vi "Bind Controls to SmartDashboard.vi"(4 "RPC ref":refnum<user-event>, 6 "Update Time (ms)":i32=100, 8 "Client Name":string="Dashboard", 9 "Path Prefix":string="SmartDashboard", 10 "Bound Control Refs":refnum<vi>[](array[refnum]), 11 "Server IP Address":string="localhost") -> ()   [LabVIEW 2017]
doc: "Place this VI in the Dashboard or other client applications so that it can run in parallel with the other tasks. Provide the robot IP address so that it can know where to find the server. This starts the NT Client automatically.\n\nCombine the path prefix and control name to construct entry names. Bind controls and indicators to a SmartDashboard or Network Table entry with the matching name. Controls and Indicators will be updated each time the table entriy of the same name changes. Table entries will be updated each time the control changes value."
uses:
  <vilib>/Rock Robotics/Network Tables/NT Event Type.ctl
  <vilib>/Rock Robotics/Network Tables/Protocol Operations.ctl
  <vilib>/Rock Robotics/Network Tables/Field Data.ctl
  <vilib>/Rock Robotics/Network Tables/Field Type.ctl
  <vilib>/Rock Robotics/Network Tables/Sequence.ctl
  <vilib>/Rock Robotics/Network Tables/NT Globals.vi
  <vilib>/Rock Robotics/WPI/Dashboard/WPI_DashboardLogging Global.vi
panel:
  in  "Finish":bool
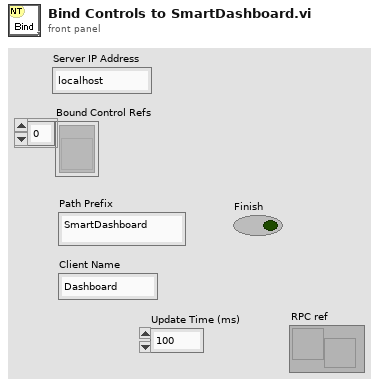
[diagram p1: front panel]
types:
  T1 = typedef "NT Event Type.ctl" = cluster{"Operation":T2, "Name":string, "Field Value":T3}
  T2 = typedef "Protocol Operations.ctl" = enum16{"Unknown", "Keep Alive", "Client Hello", "Version not supported", "Server Hello Complete", "Assign", "Update", "No Op", "Server Hello", "Client Hello Complete", "Update Flags", "Delete Entry", "Delete All", "RPC Exec", "RPC Response"}
  T3 = typedef "Field Data.ctl" = cluster{"Dbl":dbl, "String":string, "Type":T4, "Boolean":bool, "Sequence #":T5, "Flags":u8}
  T4 = typedef "Field Type.ctl" = enum8{"Invalid", "Bool", "Numeric", "String", "Raw", "Boolean Array", "Numeric Array", "String Array", "RPC"}
  T5 = typedef "Sequence.ctl" = u16
  T6 = cluster{"Operation":T2, "Name":string, "Field Value":T3}
  T7 = cluster{cluster{"RPC field ID":u16, "Unique ID":u16}, "String":string}
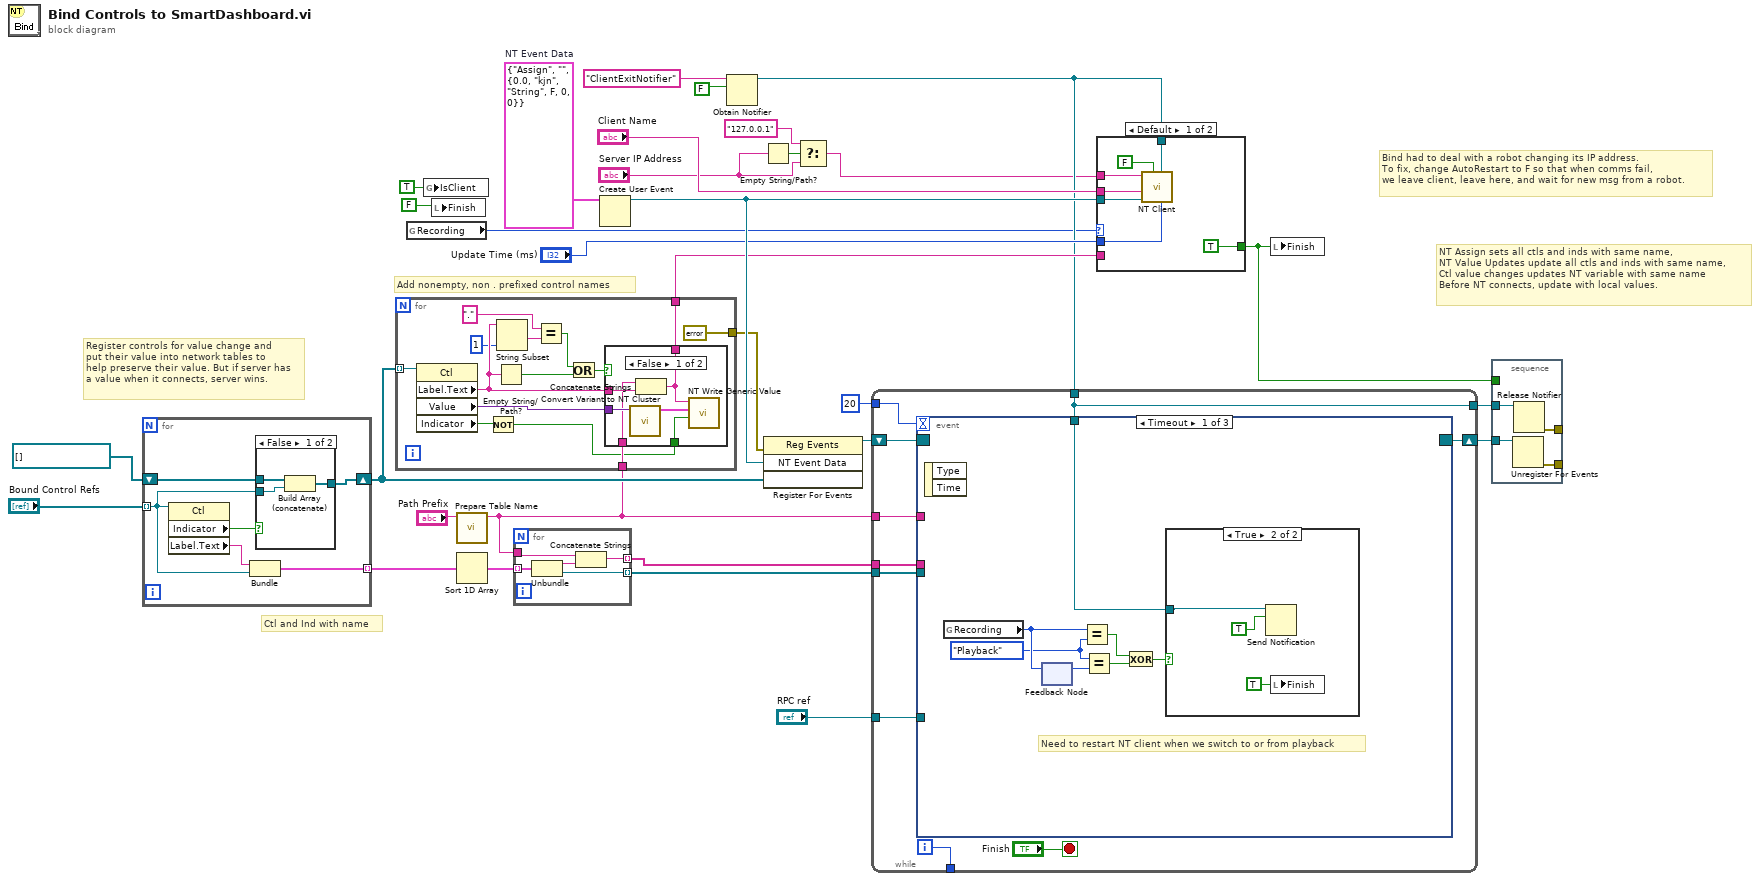
[diagram p0: block diagram]
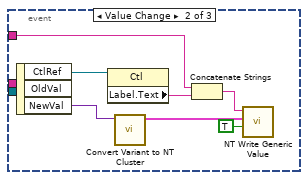
[diagram p3: hidden frame]
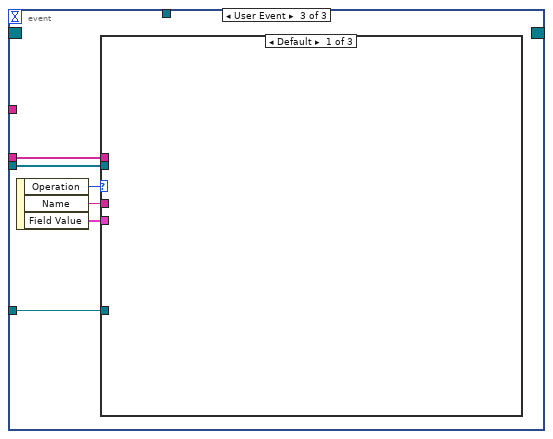
[diagram p4: hidden frame]
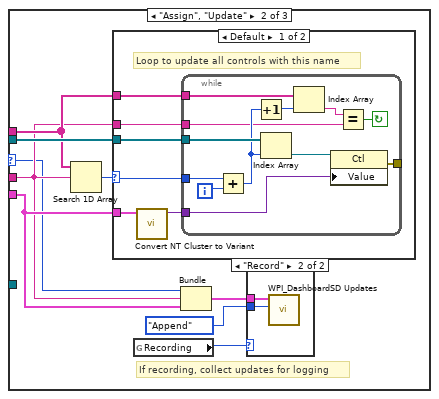
[diagram p5: hidden frame]
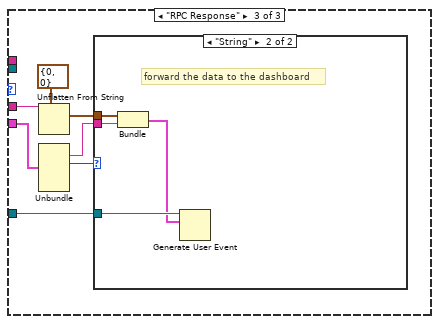
[diagram p8: hidden frame]
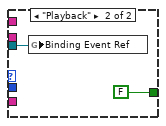
[diagram p10: hidden frame]
diagram:
  w14 = T1 {"Operation"=enum."Assign", "Name"="", "Field Value"={"Dbl"=0.0, "String"="kjn", "Type"=enum."String", "Boolean"=FALSE, "Sequence #"=0, "Flags"=0}}  # NT Event Data
  # "Add nonempty, non . prefixed control names"
  # "Bind had to deal with a robot changing its IP address.\nTo fix, change AutoRestart to F so that when comms fail,\nwe leave client, leave here, and wait for new msg from a robot."
  # "Register controls for value change and\nput their value into network tables to\nhelp preserve their value. But if server has\na value when it connects, server wins."
  # "Ctl and Ind with name"
  # "NT Assign sets all ctls and inds with same name,\nNT Value Updates update all ctls and inds with same name,\nCtl value changes updates NT variable with same name\nBefore NT connects, update with local values."
  n1 = for {
    tunnel: "Bound Control Refs" -> [w34] mode=indexing
    shift-right: [w35] -> w23
    shift-left: refnum<vi>[] [] -> [w36]
    tunnel: [w32] -> w29 mode=indexing
    n2 = property class="Ctl"(reference=w34) -> ("Indicator"=w37:bool, "Label.Text"=w33:string)  [unwired: 1 in, 2 out]
    n3 = Bundle("Label.Text"=w33, w34) -> (w32:cluster{"Label.Text":string, refnum<vi>})  [unwired: 1 in]
    n4 = case shown="False" w37 {
      tunnel: w34 -> [w40 _]
      tunnel: w36 -> [w39 w41]
      tunnel: [w38 w41] -> w35
      frame False {
        n5 = Build Array (concatenate)(w39, w40) -> (w38:refnum<vi>[])
      }
      frame True {
      }
    }
  }
  n6 = global read "WPI_DashboardLogging Global.vi" "Recording"() -> (w3:enum32{"Stop", "Record", "Playback"})
  n7 = global write "NT Globals.vi" "IsClient"(TRUE ("IsClient")) -> ()
  n8 = local write "Finish"(FALSE ("Automatic restart")) -> ()
  n9 = call <vilib>:"Prepare Table Name.vi"("Table Prefix"="Path Prefix") -> ("Prefixed Name"=w21:string)  [unwired: 10 in]
  n10 = for {
    tunnel: w23 -> [w55] mode=indexing
    tunnel: [w53] -> w24
    tunnel: w21 -> [w52]
    tunnel: [errorcluster {"status"=FALSE, "code"=0, "source"=""} ("error out")] -> w1
    n11 = property class="Ctl"(reference=w55) -> ("Label.Text"=w50:string, "Value"=w54:variant, "Indicator"=w43:bool)  [unwired: 1 in, 2 out]
    n12 = Not(x=w43) -> (.not. x?=w42:bool)
    n13 = Empty String/Path?(string/path=w50) -> (empty?=w51:bool)
    n14 = String Subset(string=w50, length (rest)=1) -> (substring=w48:string)  [unwired: 1 in]
    n15 = Equal?(x=".", y=w48) -> (x = y?=w46:bool)
    n16 = Or(x=w46, y=w51) -> (x .or. y?=w45:bool)
    n17 = case shown="False" w45 {
      tunnel: w54 -> [w60 _]
      tunnel: w50 -> [w59 _]
      tunnel: [w58 _] -> w53
      tunnel: w52 -> [w57 _]
      tunnel: w42 -> [w56 _]
      frame False {
        n18 = call <vilib>:"Convert Variant to NT Cluster.vi"("NewVal"=w60) -> ("Field Value"=w61:T3)  [unwired: 10 in]
        n19 = Concatenate Strings(w57, w59) -> (w58:string)
        n20 = call <vilib>:"NT Write Generic Value.vi"("Owning Write"=w56, "Field Value"=w61, "Name"=w58) -> ()  [unwired: 8 in, 1 out]
      }
      frame True {
      }
    }
  }
  n21 = Sort 1D Array(array=w29) -> (sorted array=w28:cluster{"Label.Text":string, refnum<vi>}[])
  n22 = for {
    tunnel: w28 -> [w66] mode=indexing
    tunnel: [w63] -> w27 mode=indexing
    tunnel: [w65] -> w26 mode=indexing
    tunnel: w21 -> [w62]
    n23 = Unbundle(w66) -> ("Label.Text"=w64:string, w65:refnum<vi>)
    n24 = Concatenate Strings(w62, w64) -> (w63:string)
  }
  n25 = Create User Event(user event datatype=w14) -> (user event=w30:refnum<user-event>)  [unwired: 1 in, 1 out]
  n26 = Obtain Notifier(name (unnamed)="ClientExitNotifier", notification data type=FALSE ("Automatic restart")) -> (notifier out=w10:refnum<notifier>)  [unwired: 2 in, 2 out]
  n27 = Empty String/Path?(string/path="Server IP Address") -> (empty?=w8:bool)
  n28 = register-events(error in=w1, w30, w23) -> (reference out=w19:refnum<event-registration>)  [unwired: 1 in, 1 out]
  n29 = Select(t="127.0.0.1" ("name (unnamed)"), s=w8, f="Server IP Address") -> (s? t:f=w7:string)
  n30 = while {
    tunnel: w27 -> [w75]
    tunnel: w26 -> [w74]
    tunnel: w21 -> [w73]
    tunnel: [w72] -> _
    shift-right: [w70] -> w17
    shift-left: w19 -> [w71]
    tunnel: w10 -> [w69]
    tunnel: [w69] -> w11
    tunnel: 20 -> [w68]
    tunnel: "RPC ref" -> [w67]
    i -> [w72]
    stop <- "Finish" stop-if-true
    n31 = event shown="[0] Timeout" {
      selector: w71 -> [_ _ _]
      dyn-events: [_ _ _] -> w70
      timeout: w68 -> [_ _ _]
      tunnel: w75 -> [_ _ w99]
      tunnel: w74 -> [_ _ w98]
      tunnel: w73 -> [_ w88 _]
      tunnel: w69 -> [w83 _ _]
      tunnel: w67 -> [_ _ w94]
      event Timeout {
        w77 = enum32{"Stop", "Record", "Playback"}."Playback" ("Recording")
        # "Need to restart NT client when we switch to or from playback"
        n32 = event-data() -> ()  [unwired: 1 in, 2 out]
        n33 = global read "WPI_DashboardLogging Global.vi" "Recording"() -> (w79:enum32{"Stop", "Record", "Playback"})
        n34 = feedback-in #1(w79) -> ()
        n35 = feedback #1() -> (w82:enum32{"Stop", "Record", "Playback"})  [unwired: 1 in]
        n36 = Equal?(x=w79, y=w77) -> (x = y?=w78:bool)
        n37 = Equal?(x=w77, y=w82) -> (x = y?=w81:bool)
        n38 = Exclusive Or(1:w81, 2:w78) -> (0:w80:bool)
        n39 = case shown="True" w80 {
          tunnel: w83 -> [_ w86]
          frame False {
          }
          frame True {
            n40 = Send Notification(notification=TRUE, notifier=w86) -> ()  [unwired: 1 in, 2 out]
            n41 = local write "Finish"(TRUE ("Finish")) -> ()
          }
        }
      }
      event Value Change {
        n42 = event-data() -> ("CtlRef"=w93:refnum<vi>, "NewVal"=w91:variant)  [unwired: 1 in, 1 out]
        n43 = property class="Ctl"(reference=w93) -> ("Label.Text"=w90:string)  [unwired: 1 in, 2 out]
        n44 = call <vilib>:"Convert Variant to NT Cluster.vi"("NewVal"=w91) -> ("Field Value"=w92:T3)  [unwired: 10 in]
        n45 = Concatenate Strings(w88, w90) -> (w89:string)
        n46 = call <vilib>:"NT Write Generic Value.vi"("Owning Write"=TRUE, "Field Value"=w92, "Name"=w89) -> ()  [unwired: 8 in, 1 out]
      }
      event User Event {
        n47 = event-data() -> ("Operation"=w97:T2, "Name"=w96:string, "Field Value"=w95:T3)  [unwired: 1 in]
        n48 = case shown="Default" w97 {
          selector: w97 -> [_ w100 _]
          tunnel: w99 -> [_ w106 _]
          tunnel: w98 -> [_ w107 _]
          tunnel: w96 -> [_ w101 w134]
          tunnel: w95 -> [_ w102 w133]
          tunnel: w94 -> [_ _ w129]
          frame Default {
          }
          frame "Assign", "Update" {
            # "If recording, collect updates for logging"
            n49 = Search 1D Array(1D array=w106, element=w101) -> (index of element=w108:i32)  [unwired: 1 in]
            n50 = case shown="Default" w108 {
              selector: w108 -> [w115 _]
              tunnel: w107 -> [w116 _]
              tunnel: w106 -> [w114 _]
              tunnel: w101 -> [w113 _]
              tunnel: w102 -> [w111 _]
              frame Default {
                # "Loop to update all controls with this name"
                n51 = call <vilib>:"Convert NT Cluster to Variant.vi"("Field Value"=w111) -> ("Variant"=w112:variant)  [unwired: 10 in]
                n52 = while {
                  tunnel: w116 -> [w128]
                  tunnel: w115 -> [w125]
                  tunnel: w114 -> [w124]
                  tunnel: w113 -> [w119]
                  tunnel: w112 -> [w118]
                  tunnel: [w117] -> _
                  i -> [w126]
                  stop <- w121 continue-if-true
                  n53 = Add(x=w125, y=w126) -> (x+y=w123:i32)
                  n54 = Increment(x=w123) -> (x+1=w122:i32)
                  n55 = Index Array(array=w128, index=w123) -> (element=w127:refnum<vi>)
                  n56 = Index Array(array=w124, index=w122) -> (element=w120:string)
                  n57 = property class="Ctl"(reference=w127, "Value"=w118) -> (error out=w117:errorcluster)  [unwired: 1 in, 1 out]
                  n58 = Equal?(x=w120, y=w119) -> (x = y?=w121:bool)
                }
              }
              frame -1 {
              }
            }
            n59 = global read "WPI_DashboardLogging Global.vi" "Recording"() -> (w103:enum32{"Stop", "Record", "Playback"})
            n60 = Bundle("Operation"=w100, "Name"=w101, "Field Value"=w102) -> (w105:T6)  [unwired: 1 in]
            n61 = case shown="\"Record\"" w103 {
              tunnel: w105 -> [_ w110]
              tunnel: enum16{"Append", "Read and Clear"}."Append" ("Operation") -> [_ w109]
              frame "Stop", Default {
              }
              frame "Record" {
                n62 = call <vilib>:"WPI_DashboardSD Updates.vi"("Operation"=w109, "Updates"=w110) -> ()  [unwired: 9 in, 1 out]
              }
            }
          }
          frame "RPC Response" {
            n63 = Unflatten From String(type=cluster{"RPC field ID":u16, "Unique ID":u16} {"RPC field ID"=0, "Unique ID"=0}, binary string=w134) -> (value=w132:cluster{"RPC field ID":u16, "Unique ID":u16})  [unwired: 3 in, 2 out]
            n64 = Unbundle(w133) -> ("String"=w131:string, "Type"=w130:T4)  [unwired: 4 out]
            n65 = case shown="\"String\"" w130 {
              tunnel: w132 -> [_ w139]
              tunnel: w131 -> [_ w138]
              tunnel: w129 -> [_ w137]
              frame "Invalid", Default {
              }
              frame "String" {
                # "forward the data to the dashboard"
                n66 = Bundle(w139, "String"=w138) -> (w136:T7)  [unwired: 1 in]
                n67 = Generate User Event(user event=w137, event data cluster=w136) -> ()  [unwired: 2 in, 2 out]
              }
            }
          }
        }
      }
    }
  }
  n68 = case shown="Default" w3 {
    tunnel: w7 -> [w146 _]
    tunnel: w30 -> [w145 w147]
    tunnel: w24 -> [_ _]
    tunnel: [TRUE ("Automatic restart") FALSE ("Automatic restart")] -> w9
    tunnel: "Client Name" -> [w142 _]
    tunnel: "Update Time (ms)" -> [w141 _]
    tunnel: w10 -> [w140 _]
    frame Default {
      n69 = call <vilib>:"NT Client.vi"("Update Time"=w141, "Cancel Ref"=w140, "Automatic restart"=FALSE, "user event ref"=w145, "Client Name"=w142, "Server IP Address"=w146) -> ()  [unwired: 6 in]
    }
    frame "Playback" {
      n70 = global write "WPI_DashboardLogging Global.vi" "Binding Event Ref"(w147) -> ()
    }
  }
  n71 = local write "Finish"(w9) -> ()
  n72 = stacked-sequence {
    tunnel: w17 -> [w152]
    tunnel: w11 -> [w151]
    tunnel: w9 -> [_]
    tunnel: [w150] -> _
    tunnel: [w149] -> _
    frame #0 {
      n73 = Unregister For Events(event registration refnum=w152) -> (error out=w149:errorcluster)  [unwired: 1 in]
      n74 = Release Notifier(notifier=w151) -> (error out=w150:errorcluster)  [unwired: 2 in, 2 out]
    }
  }
